vi "thorlabsWFS initialize.vi"(8 "error in (no error)":errorcluster) -> (0 "error out":errorcluster, 1 "Spots Y":i32, 2 "Spots X":i32, 3 "VISA Refnum out":refnum<visa-resource-name>)   [LabVIEW 2020, in "ThorlabsWFS.lvclass"]
uses:
  ThorlabsWFS.lvclass
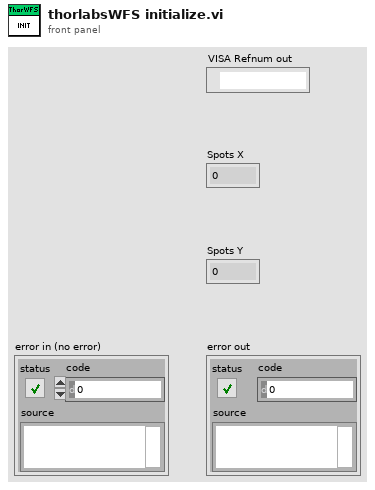
[diagram p1: front panel]
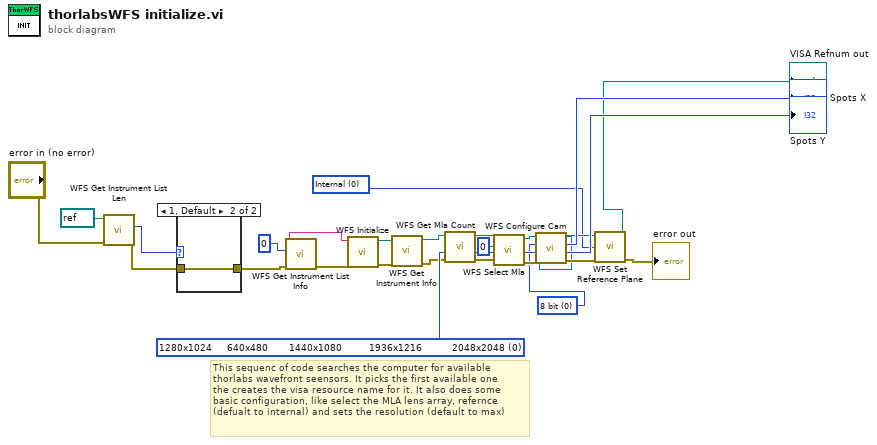
[diagram p0: block diagram]
diagram:
  w1 = 0 items=["16 bit"=1, "8 bit"=0] ("Pixel Format (8 bit)")
  w21 = 0 items=["1280x1024     640x480       1440x1080         1936x1216          2048x2048", "1024x1024     480x480       1080x1080         1216x1216          1536x1536", "768x768         360x360       768x768             1024x1024          1024x1024", "512x512         260x260       512x512             768x768              768x768    ", "320x320         180x180       360x360             512x512              512x512    ", "bin2 720x540         360x360              360x360    ", "bin2 540x540    sub2 968x608  sub2 1024x1024", "bin2 384x384    sub2 608x608      sub2 768x768", "bin2 256x256    sub2 512x512      sub2 512x512", "bin2 180x180    sub2 384x384      sub2 384x384", "sub2 256x256      sub2 256x256", "sub2 180x180      sub2 180x180"] ("Cam Resol. Index (1280x1024     640x480       1440x1080         1936x1216          2048x2048)")
  w18 = 0 items=["Internal", "User"] ("Reference Index (Internal)")
  # "This sequenc of code searches the computer for available\nthorlabs wavefront seensors. It picks the first available one\nthe creates the visa resource name for it. It also does some\nbasic configuration, like select the MLA lens array, refernce \n(defualt to internal) and sets the resolution (default to max)"
  n1 = call "WFS Get Instrument List Len.vi"("error in (no error)"="error in (no error)", "instrument handle"=refnum<visa-resource-name> refnum) -> ("error out"=w5:errorcluster, "Instrument Count"=w4:i32)  [unwired: 7 in, 1 out]
  n2 = case shown="1, Default" w4 {
    tunnel: [w27 w28] -> w6
    tunnel: w5 -> [w27 w28]
    frame 0 {
    }
    frame 1, Default {
    }
  }
  n3 = call "WFS Get Instrument List Info.vi"("error in (no error)"=w6, "Instrument List Index"=0) -> ("error out"=w8:errorcluster, "Resource Name"=w26:string)  [unwired: 3 in, 5 out]
  n4 = call "WFS Initialize.vi"("error in (no error)"=w8, "resource name"=w26) -> ("error out"=w10:errorcluster, "instrument handle out"=w9:refnum<visa-resource-name>)  [unwired: 8 in]
  n5 = call "WFS Get Instrument Info.vi"("error in (no error)"=w10, "instrument handle"=w9) -> ("error out"=w12:errorcluster, "instrument handle out"=w11:refnum<visa-resource-name>)  [unwired: 4 in, 4 out]
  n6 = call "WFS Get Mla Count.vi"("error in (no error)"=w12, "instrument handle"=w11) -> ("error out"=w14:errorcluster, "instrument handle out"=w13:refnum<visa-resource-name>)  [unwired: 7 in, 1 out]
  n7 = call "WFS Select Mla.vi"("error in (no error)"=w14, "MLA Index"=0, "instrument handle"=w13) -> ("error out"=w17:errorcluster, "instrument handle out"=w16:refnum<visa-resource-name>)  [unwired: 7 in]
  n8 = call "WFS Configure Cam.vi"("error in (no error)"=w17, "Cam Resol. Index (1280x1024     640x480       1440x1080         1936x1216          2048x2048)"=w21, "Pixel Format (8 bit)"=w1, "instrument handle"=w16) -> ("error out"=w20:errorcluster, "Spots Y"=→"Spots Y":i32, "Spots X"=→"Spots X":i32, "instrument handle out"=w19:refnum<visa-resource-name>)  [unwired: 4 in]
  n9 = call "WFS Set Reference Plane.vi"("error in (no error)"=w20, "Reference Index (Internal)"=w18, "instrument handle"=w19) -> ("error out"=→"error out":errorcluster, "instrument handle out"=→"VISA Refnum out":refnum<visa-resource-name>)  [unwired: 7 in]
